vi "Drive Straight (Jeevan Anga's conflicted copy 2013-04-07).vi"   [LabVIEW 2011]
uses:
  jeevan/Global Variables.vi
types:
  T1 = cluster{"Drive Value Output String":string, "Steer Value Output String":string, "Error Out":errorcluster}
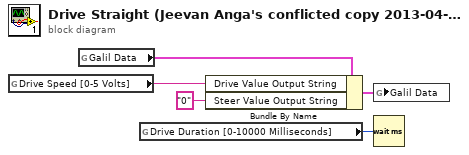
[diagram p0: block diagram]
diagram:
  n1 = global read "Global Variables.vi" "Drive Speed [0-5 Volts]"() -> (w1:string)
  n2 = global read "Global Variables.vi" "Galil Data"() -> (w4:T1)
  n3 = global read "Global Variables.vi" "Drive Duration [0-10000 Milliseconds]"() -> (w2:u32)
  n4 = Bundle By Name(cluster=w4, "Drive Value Output String"=w1, "Steer Value Output String"="0") -> (w5:T1)
  n5 = global write "Global Variables.vi" "Galil Data"(w5) -> ()
  n6 = Wait (ms)(milliseconds to wait=w2) -> ()  [unwired: 1 out]
